vi "GetFPGAData.vi"() -> ()   [LabVIEW 2017]
uses:
  <vilib>/FPGAPlugInAG/cRIO-9031/niLvFpga_Open_cRIO-9031.vi
  <vilib>/rvi/interface/common/dynamic/niFpgaDynamicAddResources.vi
  <vilib>/Utility/error.llb/Error Cluster From Error Code.vi
  <vilib>/rvi/errors/niLvFpgaAdjustHostInterfaceError.vi
  <vilib>/FPGAPlugInAG/Dynamic/niLvFpga_Close_Dynamic.vi
  <vilib>/rvi/interface/nirviOpenFPGA/nirviOpenFPGA.xnode
  FPGA Bitfiles/UMDLoopAlgCOMP2_FPGATarget_FPGAMain_LUE77PZMX6w.lvbitx
  FPGAVIs/FPGA_Main.vi
  <vilib>/rvi/interface/nirviReadWriteControl/nirviReadWriteControl.xnode
  <vilib>/rvi/interface/nirviCloseFPGA/nirviCloseFPGA.xnode
  NiFpgaLv.dll
  <vilib>/rvi/interface/Simulation/niFpgaSimulationCallBeginRW.vi
panel:
  in  "FPGA_Data":T1
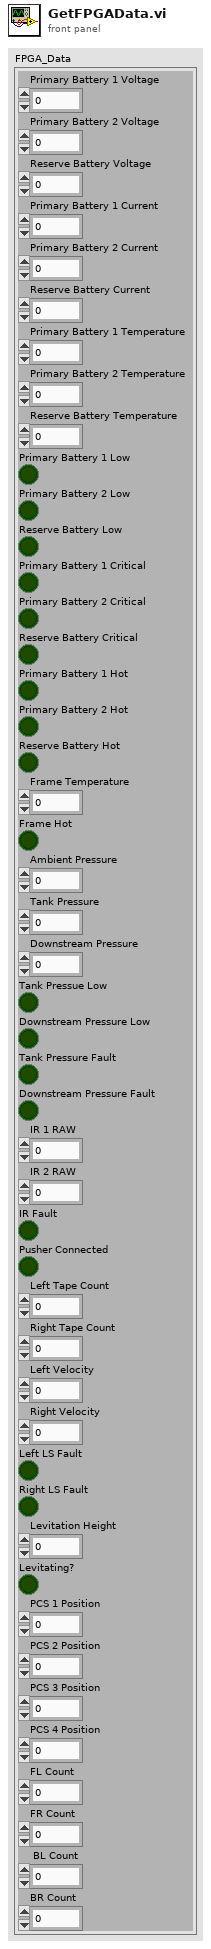
[diagram p1: front panel]
types:
  T1 = cluster{"Primary Battery 1 Voltage":sgl, "Primary Battery 2 Voltage":sgl, "Reserve Battery Voltage":sgl, "Primary Battery 1 Current":sgl, "Primary Battery 2 Current":sgl, "Reserve Battery Current":sgl, "Primary Battery 1 Temperature":sgl, "Primary Battery 2 Temperature":sgl, "Reserve Battery Temperature":sgl, "Primary Battery 1 Low":bool, "Primary Battery 2 Low":bool, "Reserve Battery Low":bool, "Primary Battery 1 Critical":bool, "Primary Battery 2 Critical":bool, "Reserve Battery Critical":bool, "Primary Battery 1 Hot":bool, "Primary Battery 2 Hot":bool, "Reserve Battery Hot":bool, "Frame Temperature":sgl, "Frame Hot":bool, "Ambient Pressure":sgl, "Tank Pressure":sgl, "Downstream Pressure":sgl, "Tank Pressue Low":bool, "Downstream Pressure Low":bool, "Tank Pressure Fault":bool, "Downstream Pressure Fault":bool, "IR 1 RAW":sgl, "IR 2 RAW":sgl, "IR Fault":bool, "Pusher Connected":bool, "Left Tape Count":u32, "Right Tape Count":u32, "Left Velocity":sgl, "Right Velocity":sgl, "Left LS Fault":bool, "Right LS Fault":bool, "Levitation Height":sgl, "Levitating?":bool, "PCS 1 Position":sgl, "PCS 2 Position":sgl, "PCS 3 Position":sgl, "PCS 4 Position":sgl, "FL Count":u8, "FR Count":u8, " BL Count":u8, "BR Count":u8}
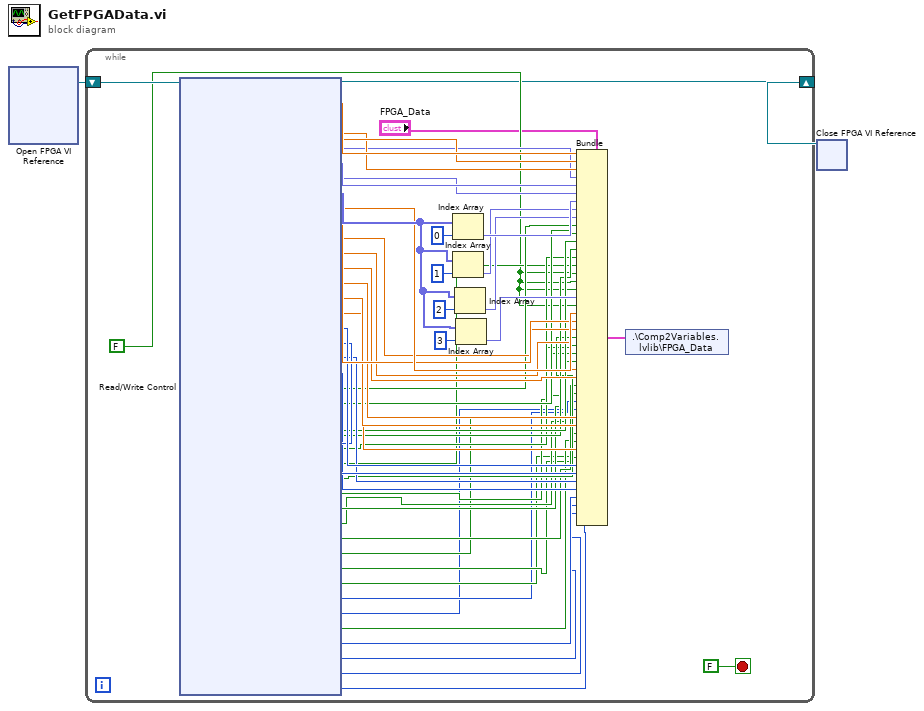
[diagram p0: block diagram]
diagram:
  n1 = xnode "Open FPGA VI Reference"() -> ("FPGA VI Reference Out"=w2:refnum<k20>)  [unwired: 2 in, 1 out]
  n2 = while {
    shift-right: [w9] -> w1
    shift-left: w2 -> [w56]
    stop <- FALSE stop-if-true
    w22 = FALSE
    n3 = xnode "Read/Write Control"("FPGA VI Reference In"=w56) -> ("FPGA VI Reference Out"=w9:refnum<k20>, "Primary Battery 1 Voltage"=w55:sgl, "Primary Battery 2 Voltage"=w54:sgl, "Reserve Battery Voltage"=w53:sgl, "Primary Battery 1 Current"=w52:fxp<+/-,55,8>, "Primary Battery 2 Current"=w51:fxp<+/-,55,8>, "Reserve Battery Current"=w50:fxp<+/-,55,8>, "TC Voltages"=w42:fxp<+/-,25,-1>[], "Ambient Pressure"=w40:sgl, "Tank Pressure"=w39:sgl, "Downstream Left Pressure"=w38:sgl, "IR 1 RAW"=w37:sgl, "IR 2 RAW"=w36:sgl, "Velocity Left (m/s)"=w35:sgl, "Velocity Right (m/s)"=w34:sgl, "Levitation Height"=w33:sgl, "PCS 1 Position"=w32:i16, "PCS 2 Position"=w31:i16, "PCS 3 Position"=w30:i16, "PCS 4 Position"=w29:i16, "Primary Battery 1 Low"=w28:bool, "Primary Battery 2 Low"=w27:bool, "Reserve Battery Low"=w26:bool, "Primary Battery 1 Critical"=w25:bool, "Primary Battery 2 Critical"=w24:bool, "Reserve Battery Critical"=w23:bool, "Tank Pressue Low"=w21:bool, "Downstream Pressure Low"=w20:bool, "Tank Pressure Fault"=w19:bool, "Downstream Pressure Fault"=w18:bool, "IR Fault"=w17:bool, "Left LS Fault"=w15:bool, "Right LS Fault"=w14:bool, "Levitating?"=w13:bool, "Left Tape Count"=w12:u32, "Right Tape Count"=w11:u32, "Pusher Connected"=w16:bool, "FL Count"=w6:u8, "FR Count"=w5:u8, "BL Count"=w4:u8, "BR Count"=w3:u8)  [unwired: 1 in, 1 out]
    n4 = Index Array(array=w42, index=0) -> (element=w49:fxp<+/-,25,-1>)
    n5 = Index Array(array=w42, index=1) -> (element=w45:fxp<+/-,25,-1>)
    n6 = Index Array(array=w42, index=2) -> (element=w44:fxp<+/-,25,-1>)
    n7 = Index Array(array=w42, index=3) -> (element=w41:fxp<+/-,25,-1>)
    n8 = Bundle(cluster="FPGA_Data", "Primary Battery 1 Voltage"=w55, "Primary Battery 2 Voltage"=w54, "Reserve Battery Voltage"=w53, "Primary Battery 1 Current"=w52, "Primary Battery 2 Current"=w51, "Reserve Battery Current"=w50, "Primary Battery 1 Temperature"=w49, "Primary Battery 2 Temperature"=w45, "Reserve Battery Temperature"=w44, "Primary Battery 1 Low"=w28, "Primary Battery 2 Low"=w27, "Reserve Battery Low"=w26, "Primary Battery 1 Critical"=w25, "Primary Battery 2 Critical"=w24, "Reserve Battery Critical"=w23, "Primary Battery 1 Hot"=w22, "Primary Battery 2 Hot"=w22, "Reserve Battery Hot"=w22, "Frame Temperature"=w41, "Frame Hot"=w22, "Ambient Pressure"=w40, "Tank Pressure"=w39, "Downstream Pressure"=w38, "Tank Pressue Low"=w21, "Downstream Pressure Low"=w20, "Tank Pressure Fault"=w19, "Downstream Pressure Fault"=w18, "IR 1 RAW"=w37, "IR 2 RAW"=w36, "IR Fault"=w17, "Pusher Connected"=w16, "Left Tape Count"=w12, "Right Tape Count"=w11, "Left Velocity"=w35, "Right Velocity"=w34, "Left LS Fault"=w15, "Right LS Fault"=w14, "Levitation Height"=w33, "Levitating?"=w13, "PCS 1 Position"=w32, "PCS 2 Position"=w31, "PCS 3 Position"=w30, "PCS 4 Position"=w29, "FL Count"=w6, "FR Count"=w5, "BL Count"=w4, "BR Count"=w3) -> (w7:T1)
    n9 = shared-variable ".\\Comp2Variables.lvlib\\FPGA_Data"(w7) -> ()  [unwired: 1 in, 1 out]
  }
  n10 = xnode "Close FPGA VI Reference"("FPGA VI Reference In"=w1) -> ()  [unwired: 1 in, 1 out]
